vi "standard deviation from power spectrum.vi"(11 "Power Spectrum":cluster{"f0":dbl, "df":dbl, "magnitude":dbl[]}) -> (3 "Numeric":dbl)   [LabVIEW 2020]
uses:
  <vilib>/Analysis/8numeric.llb/1D Numeric Integration.vi
  <vilib>/Analysis/NI_AALPro.lvlib
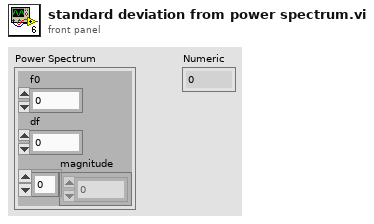
[diagram p1: front panel]
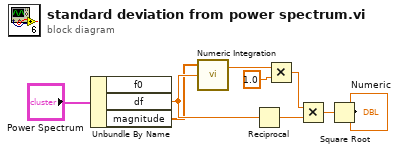
[diagram p0: block diagram]
diagram:
  n1 = Unbundle By Name("Power Spectrum") -> ("df"=w5:dbl, "magnitude"=w4:dbl[])  [unwired: 1 out]
  n2 = call-poly <vilib>:"Numeric Integration.vi"("dt"=w5, "Input Array"=w4) -> ("result"=w1:dbl)  [unwired: 1 in, 1 out]
  n3 = Reciprocal(x=w5) -> (1/x=w7:dbl)
  n4 = Multiply(x=w1, y=1.0) -> (x*y=w8:dbl)
  n5 = Multiply(x=w8, y=w7) -> (x*y=w6:dbl)
  n6 = Square Root(x=w6) -> (sqrt(x)=→"Numeric":dbl)
